vi "Module Type.vi"(11 "Config Updater Module in":refnum<class "Git Updater Module.lvclass">) -> (2 "Module Type":string)   [LabVIEW 2020, in "Volatus.lvlib" / "Git Updater Module.lvclass"]
uses:
  Git Updater Module.lvclass
  Git Updater Module.lvclass/Git Updater Module.ctl
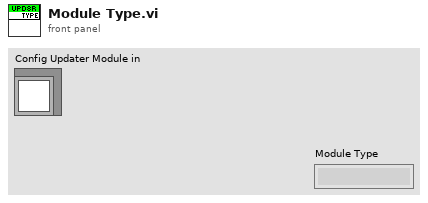
[diagram p1: front panel]
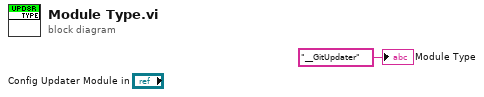
[diagram p0: block diagram]
diagram:
  "Module Type" <- "__GitUpdater" ("Module Type")
